vi "Measure.vi"(8 "error in (no error)":errorcluster caption="错误输入（无错误）", 11 "34401A 输入":refnum<class "34401A.lvclass">) -> (0 "error out":errorcluster caption="错误输出", 2 "Measurement":dbl, 3 "34401A 输出":refnum<class "34401A.lvclass">)   [LabVIEW 2020, in "34401A.lvlib" / "34401A.lvclass"]
uses:
  34401A.lvclass
  <instrlib>/Agilent 34401/Public/Data/Read (Single Point).vi
  <instrlib>/Agilent 34401/Agilent 34401.lvlib
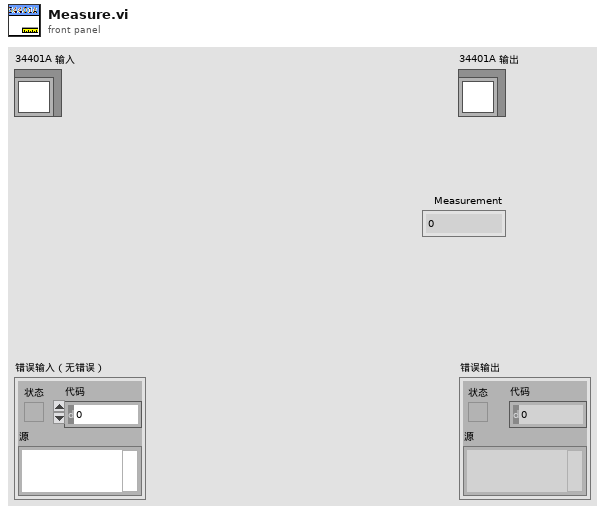
[diagram p1: front panel]
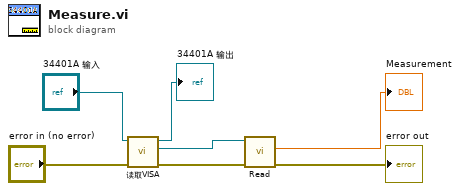
[diagram p0: block diagram]
diagram:
  n1 = call "读取VISA.vi"("error in (no error)"="error in (no error)", "数字多用表接口输入"="34401A 输入") -> ("error out"=w1:errorcluster, "VISA"=w6:refnum<visa-resource-name>, "数字多用表接口输出"=→"34401A 输出":refnum<class "34401A.lvclass">)  [unwired: 7 in]
  n2 = call-poly <instrlib>:"Read.vi"("error in (no error)"=w1, "VISA resource name"=w6) -> ("error out"=→"error out":errorcluster, "Measurement"=→"Measurement":dbl)  [unwired: 7 in, 1 out]
